vi "asset.get_from_datasouce.vi"(8 "error in":errorcluster, 10 "Datasource RID":string, 11 "Nominal Client in":refnum<class "Nominal Client.lvclass">) -> (0 "error out":errorcluster, 2 "Assets":refnum<class "asset.lvclass">[](array[class]), 3 "Nominal Client out":refnum<class "Nominal Client.lvclass">)   [LabVIEW 2020, in "Nominal Client.lvclass"]
doc: "Returns all assets with given data source as a data scope."
uses:
  Nominal Client.lvclass
  asset/asset.lvclass
  Nominal Client.lvclass/Nominal Client.ctl
  <vilib>/JDP Science/JSONtext/JSONtext.lvlib
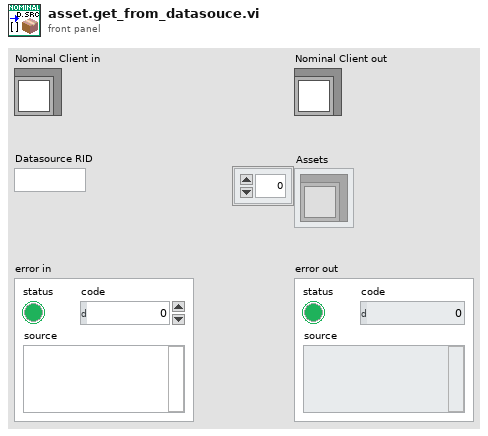
[diagram p1: front panel]
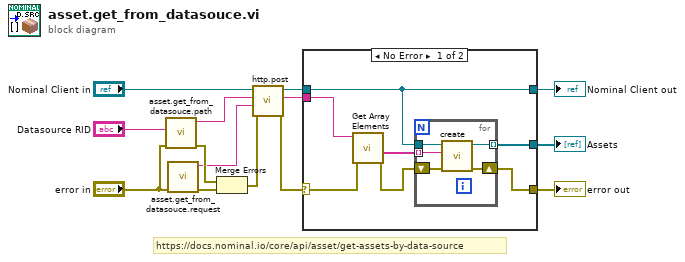
[diagram p0: block diagram]
diagram:
  # "https://docs.nominal.io/core/api/asset/get-assets-by-data-source"
  n1 = call "asset.get_from_datasouce.path.vi"("error in"="error in", "datasource rid"="Datasource RID") -> ("error out"=w4:errorcluster, "path"=w6:string)  [unwired: 8 in]
  n2 = call "asset.get_from_datasouce.request.vi"("error in"="error in") -> ("error out"=w3:errorcluster, "request"=w1:string)  [unwired: 9 in]
  n3 = Merge Errors(w4, w3) -> (w2:errorcluster)
  n4 = call "http.post.vi"("error in"=w2, "Request body"=w1, "Path"=w6, "Nominal Client in"="Nominal Client in") -> ("error out"=w9:errorcluster, "Response"=w14:string, "Nominal Client out"=w12:refnum<class "Nominal Client.lvclass">)  [unwired: 4 in, 1 out]
  n5 = case shown="No Error" w9 {
    selector: w9 -> [w18 w28]
    tunnel: w14 -> [w15 _]
    tunnel: w12 -> [w19 w27]
    tunnel: [w19 w27] -> w11
    tunnel: [w21 _] -> w10
    tunnel: [w20 w28] -> w8
    frame No Error {
      n6 = call <vilib>:"Get Array Elements.vi"("error in (no error)"=w18, "JSON"=w15) -> ("error out"=w17:errorcluster, "<JSON>"=w16:string[])  [unwired: 7 in, 1 out]
      n7 = for {
        tunnel: w16 -> [w26] mode=indexing
        tunnel: [w25] -> w21 mode=indexing
        shift-right: [w23] -> w20
        shift-left: w17 -> [w24]
        tunnel: w19 -> [w22]
        n8 = call "create.vi"("error in"=w24, "asset"=w26, "Nominal Client"=w22) -> ("error out"=w23:errorcluster, "asset"=w25:refnum<class "asset.lvclass">)  [unwired: 7 in]
      }
    }
    frame Error {
    }
  }
  "Nominal Client out" <- w11
  "error out" <- w8
  "Assets" <- w10
